vi "Strafe_Correction.vi"(8 "error in":errorcluster) -> ()   [LabVIEW 2017]
uses:
  <vilib>/Rock Robotics/Network Tables/NT Read Number.vi
  <vilib>/addons/control/pid/pid.llb/PID (DBL).vi
  <vilib>/addons/control/pid/NI_PID_pid.lvlib
panel:
  # ".035"
  # "0"
  # ".002"
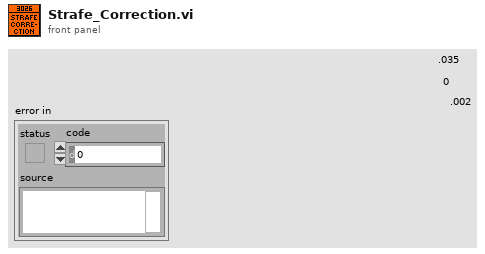
[diagram p1: front panel]
types:
  T1 = cluster{"proportional gain (Kc)":dbl, "integral time (Ti, min)":dbl, "derivative time (Td, min)":dbl}
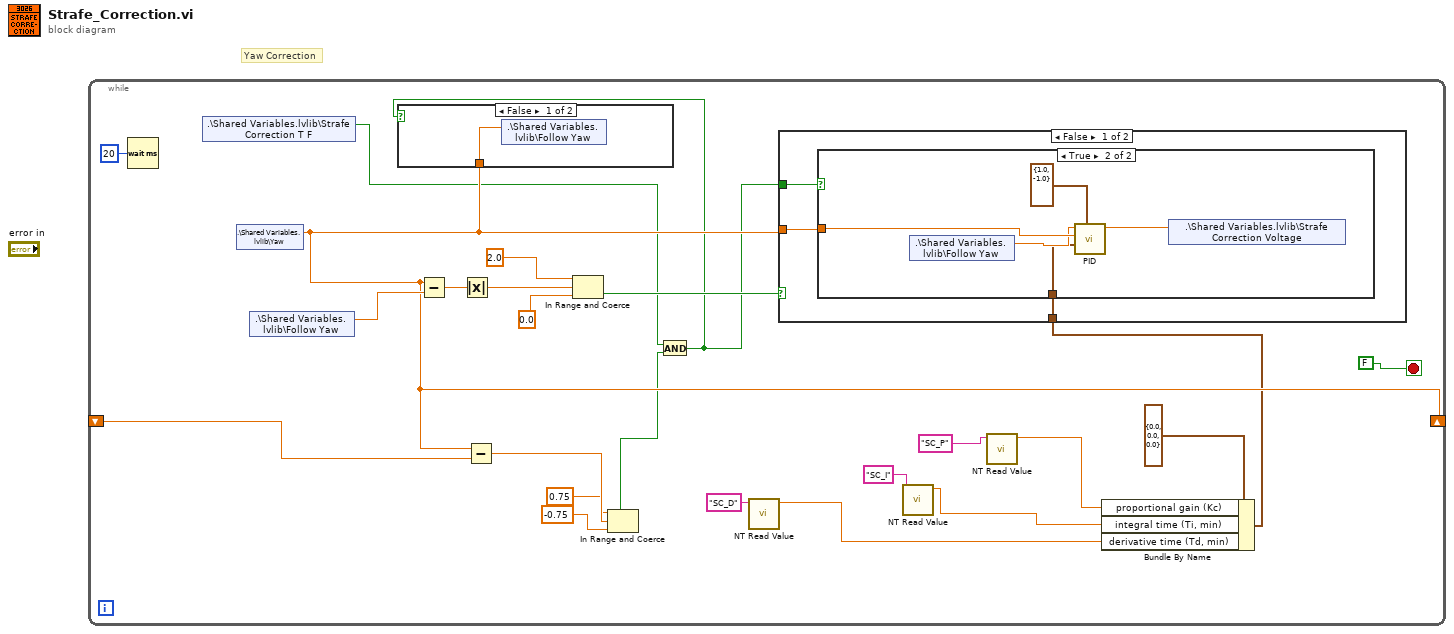
[diagram p0: block diagram]
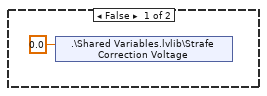
[diagram p3: hidden frame]
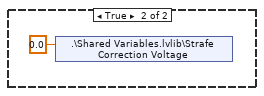
[diagram p4: hidden frame]
diagram:
  # "Yaw Correction"
  n1 = while {
    shift-right: [w16] -> _
    shift-left: _ -> [w15]
    stop <- FALSE stop-if-true
    n2 = Wait (ms)(milliseconds to wait=u32 20) -> ()  [unwired: 1 out]
    n3 = shared-variable ".\\Shared Variables.lvlib\\Strafe Correction T F"() -> (w14:bool)  [unwired: 1 in, 1 out]
    n4 = shared-variable ".\\Shared Variables.lvlib\\Yaw"() -> (w16:dbl)  [unwired: 1 in, 1 out]
    n5 = shared-variable ".\\Shared Variables.lvlib\\Follow Yaw"() -> (w22:dbl)  [unwired: 1 in, 1 out]
    n6 = Subtract(x=w16, y=w22) -> (x-y=w19:dbl)
    n7 = Absolute Value(x=w19) -> (abs(x)=w18:dbl)
    n8 = Subtract(x=w16, y=w15) -> (x-y=w11:dbl)
    n9 = In Range and Coerce(upper limit=2.0, x=w18, lower limit=0.0) -> (In Range?=w20:bool)  [unwired: 1 out]
    n10 = In Range and Coerce(upper limit=0.75, x=w11, lower limit=-0.75) -> (In Range?=w12:bool)  [unwired: 1 out]
    n11 = And(x=w14, y=w12) -> (x .and. y?=w13:bool)
    n12 = case shown="False" w13 {
      tunnel: w16 -> [w25 _]
      frame False {
        n13 = shared-variable ".\\Shared Variables.lvlib\\Follow Yaw"(w25) -> ()  [unwired: 1 in, 1 out]
      }
      frame True {
      }
    }
    n14 = call-poly <vilib>:"NT Read Value.vi"("Name"="SC_D") -> ("Numeric"=w7:dbl)  [unwired: 9 in, 1 out]
    n15 = call-poly <vilib>:"NT Read Value.vi"("Name"="SC_I") -> ("Numeric"=w8:dbl)  [unwired: 9 in, 1 out]
    n16 = call-poly <vilib>:"NT Read Value.vi"("Name"="SC_P") -> ("Numeric"=w3:dbl)  [unwired: 9 in, 1 out]
    n17 = Bundle By Name(cluster=T1 {"proportional gain (Kc)"=0.0, "integral time (Ti, min)"=0.0, "derivative time (Td, min)"=0.0} ("PID gains"), "proportional gain (Kc)"=w3, "integral time (Ti, min)"=w8, "derivative time (Td, min)"=w7) -> (w1:T1)
    n18 = case shown="False" w20 {
      tunnel: w16 -> [w28 _]
      tunnel: w13 -> [w27 _]
      tunnel: w1 -> [w26 _]
      frame False {
        n19 = case shown="True" w27 {
          tunnel: w28 -> [_ w33]
          tunnel: w26 -> [_ w30]
          frame False {
            n20 = shared-variable ".\\Shared Variables.lvlib\\Strafe Correction Voltage"(0.0 ("Strafe Correction Voltage")) -> ()  [unwired: 1 in, 1 out]
          }
          frame True {
            n21 = shared-variable ".\\Shared Variables.lvlib\\Follow Yaw"() -> (w32:dbl)  [unwired: 1 in, 1 out]
            n22 = call-poly <vilib>:"PID.vi"("output range"=cluster{"output high":dbl, "output low":dbl} {"output high"=1.0, "output low"=-1.0}, "PID gains"=w30, "process variable"=w33, "setpoint"=w32) -> ("output"=w34:dbl)  [unwired: 6 in, 1 out]
            n23 = shared-variable ".\\Shared Variables.lvlib\\Strafe Correction Voltage"(w34) -> ()  [unwired: 1 in, 1 out]
          }
        }
      }
      frame True {
        n24 = shared-variable ".\\Shared Variables.lvlib\\Strafe Correction Voltage"(0.0 ("Strafe Correction Voltage")) -> ()  [unwired: 1 in, 1 out]
      }
    }
  }
